vi "sub_ui-usertype.vi"(7 "Disabled":T1(ring)=enum."Disabled and Grayed Out") -> ()   [LabVIEW 2019]
uses:
  _ctrl/rw.ctl
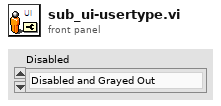
[diagram p1: front panel]
types:
  T1 = enum8{"Enabled", "Disabled", "Disabled and Grayed Out"}
  T2 = typedef "rw.ctl" = enum16{"read", "write"}
  T3 = typedef "ref_all.ctl" = cluster{"BP4610 Config":refnum<vi>, "DSP1950 Config":refnum<vi>, "2470-config":refnum<vi>, "cDAQ 9269 AO config":refnum<vi>, "cDAQ 9221 Config":refnum<vi>, "cDAQ-9467 Config":refnum<vi>, "Waveform":refnum<vi>, "DL950 wfm":refnum<vi>, "AI Graph":refnum<vi>, "AO_Wave-config":refnum<vi>, "DL950 items":refnum<vi>, "Volt":refnum<vi>, "Current":refnum<vi>, "AO_Level":refnum<vi>, "RC-Test Judgement ":refnum<vi>, "Log path":refnum<vi>, "시험명":refnum<vi>, "file renew[Hr]":refnum<vi>, "Breakdown-Spec":refnum<vi>, "paste":refnum<vi>, "copy":refnum<vi>, "DL950_config":refnum<vi>, "종료시간":refnum<vi>, "경과시간":refnum<vi>, "Apply":refnum<vi>, "DSP Config LV ":refnum<vi>, "Testconfig":refnum<vi>}
  T4 = typedef "ui_dev-operator.ctl" = cluster{"Operation stutus":refnum<vi>, "Test Status":refnum<vi>, "Setting":refnum<vi>, "Manual":refnum<vi>, "Main":refnum<vi>, "RCstart":refnum<vi>, "채널선택":refnum<vi>, "시험명":refnum<vi>, "Tab Control_manual":refnum<vi>, "시험 모드":refnum<vi>, "HW check":refnum<vi>, "login":refnum<vi>, "logout":refnum<vi>}
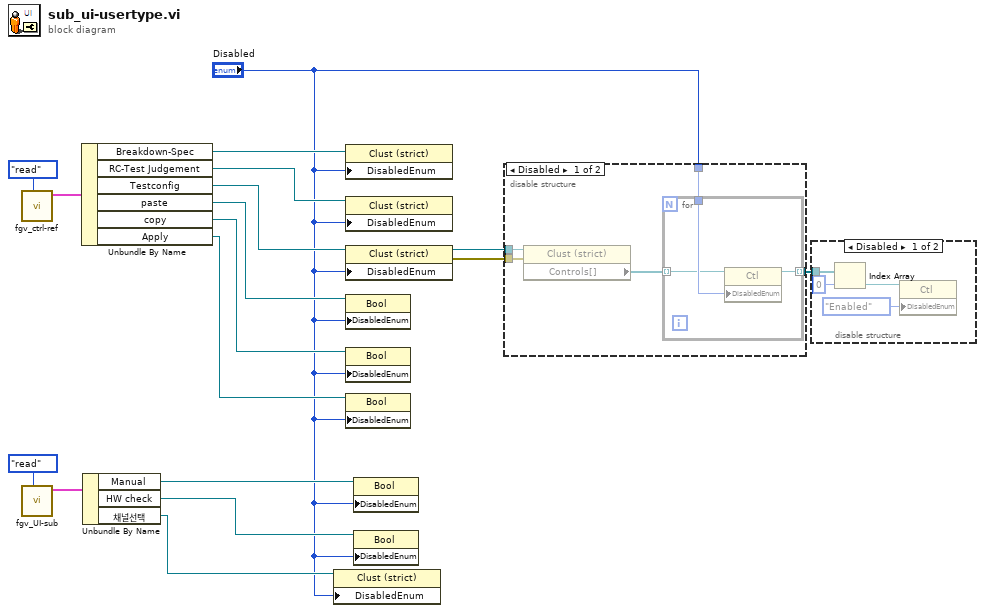
[diagram p0: block diagram]
diagram:
  n1 = call "fgv_ctrl-ref.vi"("cmd"=rw."read") -> ("output cluster 2"=w14:T3)  [unwired: 9 in, 1 out]
  n2 = call "fgv_UI-sub.vi"("cmd"=rw."read") -> ("output cluster 2"=w9:T4)  [unwired: 9 in, 1 out]
  n3 = Unbundle By Name(w14) -> ("Breakdown-Spec"=w15:refnum<vi>, "RC-Test Judgement"=w16:refnum<vi>, "Testconfig"=w17:refnum<vi>, "paste"=w12:refnum<vi>, "copy"=w11:refnum<vi>, "Apply"=w5:refnum<vi>)
  n4 = Unbundle By Name(w9) -> ("Manual"=w8:refnum<vi>, "HW check"=w7:refnum<vi>, "채널선택"=w6:refnum<vi>)
  n5 = property class="Clust (strict)"(reference=w6, "DisabledEnum"="Disabled") -> ()  [unwired: 1 in, 2 out]
  n6 = property class="Clust (strict)"(reference=w15, "DisabledEnum"="Disabled") -> ()  [unwired: 1 in, 2 out]
  n7 = property class="Clust (strict)"(reference=w16, "DisabledEnum"="Disabled") -> ()  [unwired: 1 in, 2 out]
  n8 = property class="Clust (strict)"(reference=w17, "DisabledEnum"="Disabled") -> (reference out=w4:refnum<vi>, error out=w3:errorcluster)  [unwired: 1 in]
  n9 = property class="Bool"(reference=w12, "DisabledEnum"="Disabled") -> ()  [unwired: 1 in, 2 out]
  n10 = property class="Bool"(reference=w11, "DisabledEnum"="Disabled") -> ()  [unwired: 1 in, 2 out]
  n11 = property class="Bool"(reference=w5, "DisabledEnum"="Disabled") -> ()  [unwired: 1 in, 2 out]
  n12 = property class="Bool"(reference=w8, "DisabledEnum"="Disabled") -> ()  [unwired: 1 in, 2 out]
  n13 = property class="Bool"(reference=w7, "DisabledEnum"="Disabled") -> ()  [unwired: 1 in, 2 out]
  n14 = disable-structure shown="Disabled" {
    disable-tunnel: w4 -> [w22 _]
    disable-tunnel: w3 -> [w21 _]
    disable-tunnel: [w19 _] -> w2
    disable-tunnel: "Disabled" -> [w18 _]
    frame Disabled {
      n15 = property class="Clust (strict)"(reference=w22, error in=w21) -> ("Controls[]"=w20:refnum<vi>[])  [unwired: 2 out]
      n16 = for {
        tunnel: w18 -> [w25]
        tunnel: w20 -> [w24] mode=indexing
        tunnel: [w23] -> w19 mode=indexing
        n17 = property class="Ctl"(reference=w24, "DisabledEnum"=w25) -> (reference out=w23:refnum<vi>)  [unwired: 1 in, 1 out]
      }
    }
    frame Enabled {
    }
  }
  n18 = disable-structure shown="Disabled" {
    disable-tunnel: w2 -> [w29 _]
    frame Disabled {
      n19 = Index Array(array=w29, index=0) -> (element=w28:refnum<vi>)
      n20 = property class="Ctl"(reference=w28, "DisabledEnum"=T1."Enabled" ("Disabled")) -> ()  [unwired: 1 in, 2 out]
    }
    frame Enabled {
    }
  }
